vi "SVT Hydrodynamic Journal Bearing.vi"(0 "nominal speed [RPM]":dbl=1200.0 min=0.0, 5 "oil whirl order":dbl=0.45, 11 "error in (no error)":errorcluster) -> (4 "oil whirl frequency":dbl=9.0, 15 "error out":errorcluster)   [LabVIEW 2017, in "SoundVib_MachineCharacteristic.lvlib"]
doc: "Calculates characteristic frequencies or orders of rolling-element bearings or hydrodynamic journal bearings. You must manually select the polymorphic instance you want to use."
uses:
  <vilib>/addons/Sound and Vibration/svt_Machine Characteristic/SoundVib_MachineCharacteristic.lvlib
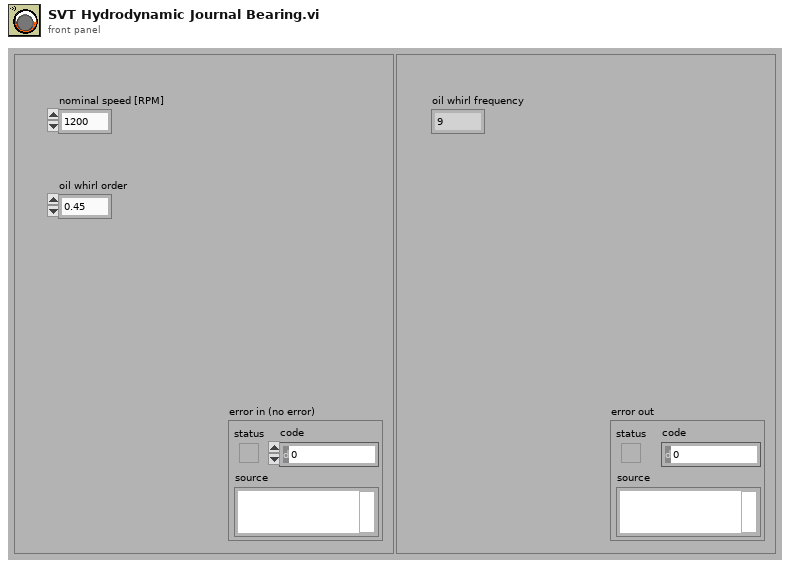
[diagram p1: front panel]
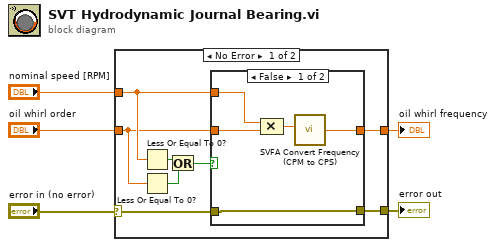
[diagram p0: block diagram]
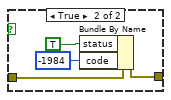
[diagram p2: hidden frame]
diagram:
  n1 = case shown="No Error" "error in (no error)" {
    selector: "error in (no error)" -> [w10 w23]
    tunnel: [w9 w23] -> w4
    tunnel: "oil whirl order" -> [w7 _]
    tunnel: "nominal speed [RPM]" -> [w8 _]
    tunnel: [w6 _] -> w1
    frame No Error {
      n2 = Less Or Equal To 0?(x=w8) -> (x <= 0?=w13:bool)
      n3 = Less Or Equal To 0?(x=w7) -> (x <= 0?=w12:bool)
      n4 = Or(x=w13, y=w12) -> (x .or. y?=w11:bool)
      n5 = case shown="False" w11 {
        tunnel: w10 -> [w18 w22]
        tunnel: [w18 w21] -> w9
        tunnel: w8 -> [w17 _]
        tunnel: w7 -> [w16 _]
        tunnel: [w14 _] -> w6
        frame False {
          n6 = Compound Arithmetic op=MULTIPLY(w17, w16) -> (w15:dbl)
          n7 = call <vilib>:"SVFA Convert Frequency (CPM to CPS).vi"("nominal speed [RPM]"=w15) -> ("frequency [Hz]"=w14:dbl)  [unwired: 5 in]
        }
        frame True {
          n8 = Bundle By Name(cluster=w22, "status"=TRUE, "code"=-1984) -> (w21:errorcluster)
        }
      }
    }
    frame Error {
    }
  }
  "error out" <- w4
  "oil whirl frequency" <- w1
